vi "CAN_controlMode.vi"(8 "error in (no error)":errorcluster, 10 "Control Mode":T2, 11 "Cluster":T4={"CAN Jaguar Ref"={"Device Number"=0, "Control Mode"=enum."Percent VBus", "Inverted"=FALSE, "Semaphore"=refnum, "Max Vout"=12.0, "DevStatus"={"status"=FALSE, "code"=0, "source"=""}}, "CAN Jaguar Ref 2"={"Device Number"=0, "Control Mode"=enum."Percent VBus", "Inverted"=FALSE, "Semaphore"=refnum, "Max Vout"=12.0, "DevStatus"={"status"=FALSE, "code"=0, "source"=""}}}) -> (0 "error out":errorcluster, 3 "output cluster":T5)   [LabVIEW 2009, in "OWNCAN.lvlib"]
uses:
  OWNCAN.lvlib
  CAN.lvlib
  CAN/SubVIs/CAN Jaguar Control Mode.ctl
  CAN/SubVIs/CAN Jaguar Ref.ctl
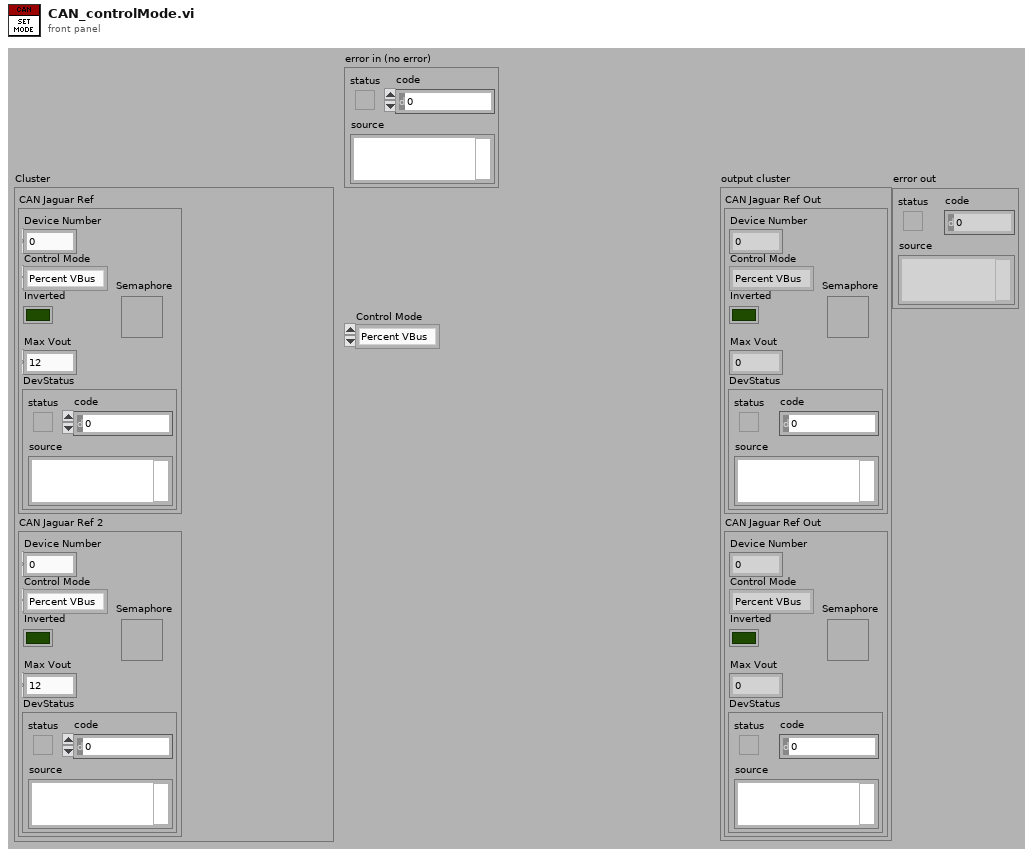
[diagram p1: front panel]
types:
  T1 = typedef "CAN.lvlib/CAN Jaguar Ref.ctl" = cluster{"Device Number":u8, "Control Mode":T2, "Inverted":bool, "Semaphore":T3, "Max Vout":dbl, "DevStatus":errorcluster}
  T2 = typedef "CAN.lvlib/CAN Jaguar Control Mode.ctl" = enum16{"Percent VBus", "Speed", "Position", "Current"}
  T3 = typedef "Semaphore RefNum" = refnum<k1>
  T4 = cluster{"CAN Jaguar Ref":T1, "CAN Jaguar Ref 2":T1}
  T5 = cluster{"CAN Jaguar Ref Out":T1, "CAN Jaguar Ref Out":T1}
  T6 = cluster{"PID Position":cluster{"P":dbl, "I":dbl, "D":dbl}, "PID Position 2":cluster{"P":dbl, "I":dbl, "D":dbl}}
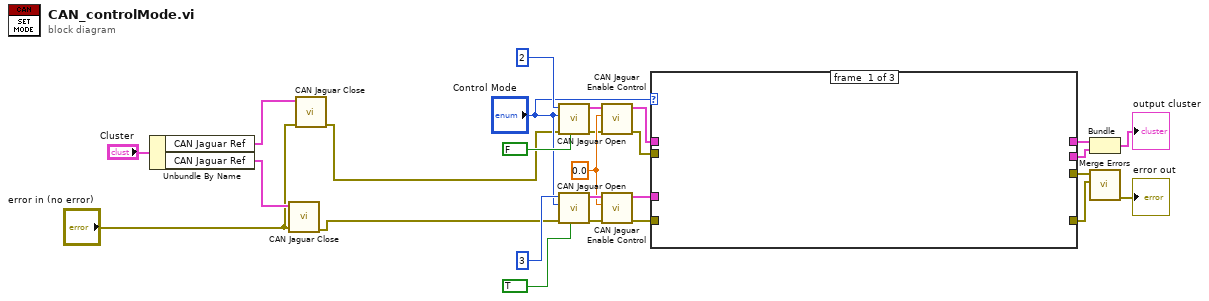
[diagram p0: block diagram]
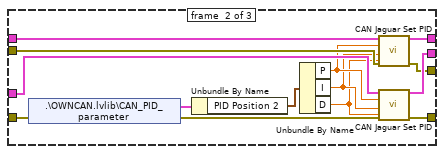
[diagram p2: hidden frame]
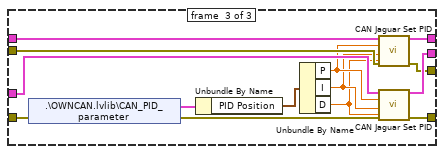
[diagram p3: hidden frame]
diagram:
  w20 = 0.0 ("Encoder Initial Position")
  n1 = Unbundle By Name("Cluster") -> ("CAN Jaguar Ref"=w5:T1, "CAN Jaguar Ref"=w4:T1)
  n2 = call "CAN Jaguar Close.vi"("error in (no error)"="error in (no error)", "CAN Jaguar Ref"=w4) -> ("error out"=w1:errorcluster)  [unwired: 9 in]
  n3 = call "CAN Jaguar Close.vi"("error in (no error)"="error in (no error)", "CAN Jaguar Ref"=w5) -> ("error out"=w2:errorcluster)  [unwired: 9 in]
  n4 = call "CAN Jaguar Open.vi"("Inverted"=FALSE, "error in (no error)"=w2, "Control Mode"="Control Mode", "Device Number"=u8 2) -> ("error out"=w19:errorcluster, "CAN Jaguar Ref Out"=w17:T1)  [unwired: 6 in]
  n5 = call "CAN Jaguar Open.vi"("Inverted"=TRUE, "error in (no error)"=w1, "Control Mode"="Control Mode", "Device Number"=u8 3) -> ("error out"=w18:errorcluster, "CAN Jaguar Ref Out"=w21:T1)  [unwired: 6 in]
  n6 = call "CAN Jaguar Enable Control.vi"("error in (no error)"=w19, "Encoder Initial Position"=w20, "CAN Jaguar Ref"=w17) -> ("error out"=w14:errorcluster, "CAN Jaguar Ref Out"=w13:T1)  [unwired: 7 in]
  n7 = call "CAN Jaguar Enable Control.vi"("error in (no error)"=w18, "Encoder Initial Position"=w20, "CAN Jaguar Ref"=w21) -> ("error out"=w11:errorcluster, "CAN Jaguar Ref Out"=w12:T1)  [unwired: 7 in]
  n8 = case shown="\"Percent VBus\", Default" "Control Mode" {
    tunnel: w14 -> [_ w40 w54]
    tunnel: w13 -> [_ w39 w53]
    tunnel: w12 -> [_ w38 w52]
    tunnel: w11 -> [_ w32 w46]
    tunnel: [_ w37 w51] -> w10
    tunnel: [_ w36 w50] -> w9
    tunnel: [_ w35 w49] -> w8
    tunnel: [_ w34 w48] -> w7
    frame #0 {
    }
    frame #1 {
      n9 = shared-variable ".\\OWNCAN.lvlib\\CAN_PID_parameter"(error in=w32) -> (w33:T6, error out=w31:errorcluster)
      n10 = Unbundle By Name(w33) -> ("PID Position 2"=w30:cluster{"P":dbl, "I":dbl, "D":dbl})
      n11 = Unbundle By Name(w30) -> ("P"=w29:dbl, "I"=w28:dbl, "D"=w27:dbl)
      n12 = call "CAN Jaguar Set PID.vi"("CAN Jaguar Ref"=w39, "P"=w29, "I"=w28, "D"=w27, "error in (no error)"=w40) -> ("CAN Jaguar Ref Out"=w36:T1, "error out"=w35:errorcluster)  [unwired: 9 in]
      n13 = call "CAN Jaguar Set PID.vi"("CAN Jaguar Ref"=w38, "P"=w29, "I"=w28, "D"=w27, "error in (no error)"=w31) -> ("CAN Jaguar Ref Out"=w37:T1, "error out"=w34:errorcluster)  [unwired: 9 in]
    }
    frame #2 {
      n14 = shared-variable ".\\OWNCAN.lvlib\\CAN_PID_parameter"(error in=w46) -> (w47:T6, error out=w45:errorcluster)
      n15 = Unbundle By Name(w47) -> ("PID Position"=w44:cluster{"P":dbl, "I":dbl, "D":dbl})
      n16 = Unbundle By Name(w44) -> ("P"=w43:dbl, "I"=w42:dbl, "D"=w41:dbl)
      n17 = call "CAN Jaguar Set PID.vi"("CAN Jaguar Ref"=w53, "P"=w43, "I"=w42, "D"=w41, "error in (no error)"=w54) -> ("CAN Jaguar Ref Out"=w50:T1, "error out"=w49:errorcluster)  [unwired: 9 in]
      n18 = call "CAN Jaguar Set PID.vi"("CAN Jaguar Ref"=w52, "P"=w43, "I"=w42, "D"=w41, "error in (no error)"=w45) -> ("CAN Jaguar Ref Out"=w51:T1, "error out"=w48:errorcluster)  [unwired: 9 in]
    }
  }
  n19 = Bundle("CAN Jaguar Ref Out"=w9, "CAN Jaguar Ref Out"=w10) -> (→"output cluster":T5)  [unwired: 1 in]
  n20 = call <vilib>:"Merge Errors.vi"("error in 2 (no error)"=w7, "error in 1 (no error)"=w8) -> ("error out"=→"error out":errorcluster)  [unwired: 5 in]
